vi "Verify Trim toque 4.vi"(6 "error in":errorcluster, 8 "MaxRead":i32, 9 "Channel in":u16) -> (0 "error out":errorcluster, 1 "Messages":T1(array[cluster]), 2 "Pass":bool, 3 "Channel out":u16)   [LabVIEW 2023]
uses:
  daf79331-edb1-4423-8e39-327e2c4704bb.vi
  Communication/PCAN2023/PCAN API.lvlib
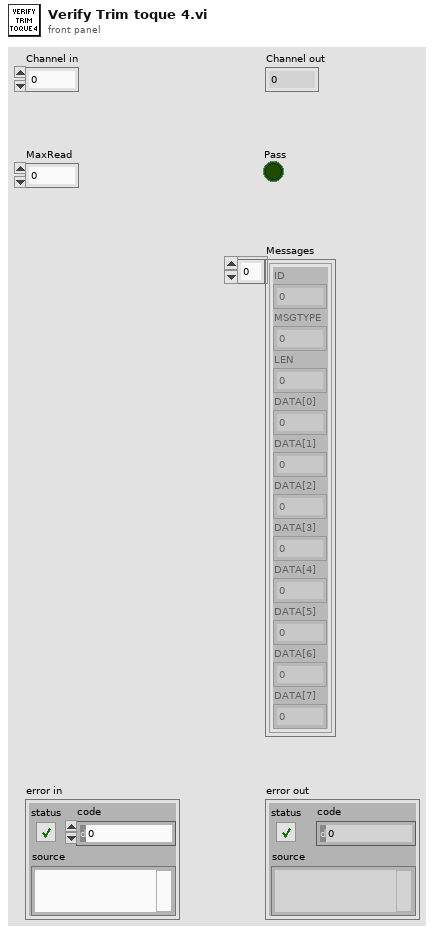
[diagram p1: front panel]
types:
  T1 = cluster{"ID":u32, "MSGTYPE":u8, "LEN":u8, "DATA[0]":u8, "DATA[1]":u8, "DATA[2]":u8, "DATA[3]":u8, "DATA[4]":u8, "DATA[5]":u8, "DATA[6]":u8, "DATA[7]":u8}[]
  T2 = cluster{"ID":u32, "MSGTYPE":u8, "LEN":u8, "DATA[0]":u8, "DATA[1]":u8, "DATA[2]":u8, "DATA[3]":u8, "DATA[4]":u8, "DATA[5]":u8, "DATA[6]":u8, "DATA[7]":u8}
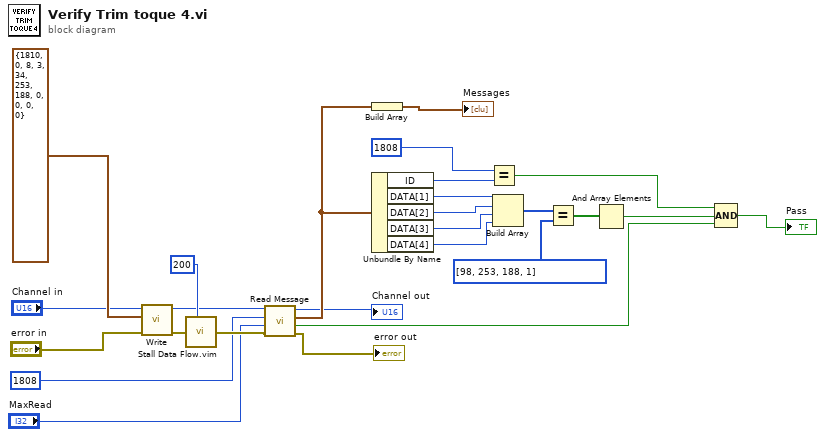
[diagram p0: block diagram]
diagram:
  n1 = call "Write.vi"("error in"="error in", "MessageBuffer"=T2 {"ID"=1810, "MSGTYPE"=0, "LEN"=8, "DATA[0]"=3, "DATA[1]"=34, "DATA[2]"=253, "DATA[3]"=188, "DATA[4]"=0, "DATA[5]"=0, "DATA[6]"=0, "DATA[7]"=0}, "Channel"="Channel in") -> ("error out"=w25:errorcluster, "Channel out"=w8:u16)  [unwired: 5 in, 2 out]
  n2 = call "Stall Data Flow.vim"("value in"=w25, "milliseconds to wait"=u32 200) -> ("value out"=w7:errorcluster)  [unwired: 1 out]
  n3 = call "Read Message.vi"("error in"=w7, "MaxRead"="MaxRead", "ID"=u32 1808, "Channel in"=w8) -> ("error out"=→"error out":errorcluster, "Passed"=w1:bool, "Last Message"=w5:T2, "Channel out"=→"Channel out":u16)  [unwired: 3 in, 1 out]
  n4 = Build Array(w5) -> (→"Messages":T1)
  n5 = Unbundle By Name(w5) -> ("ID"=w17:u32, "DATA[1]"=w21:u8, "DATA[2]"=w20:u8, "DATA[3]"=w19:u8, "DATA[4]"=w18:u8)
  n6 = Equal?(x=u32 1808, y=w17) -> (x = y?=w13:bool)
  n7 = Build Array(w21, w20, w19, w18) -> (w15:u8[])
  n8 = Equal?(x=w15, y=u8[] [98, 253, 188, 1]) -> (x = y?=w12:bool[])
  n9 = And Array Elements(Boolean array=w12) -> (logical AND=w11:bool)
  n10 = Compound Arithmetic op=AND(w13, w11, w1) -> (→"Pass":bool)
